vi "AVS Names to List.vi"(8 "error in":errorcluster, 11 "AVS names":T1) -> (0 "error out":errorcluster, 3 "List":string)   [LabVIEW 2019, in "Inst.TC.lvclass"]
uses:
  Inst.TC.lvclass
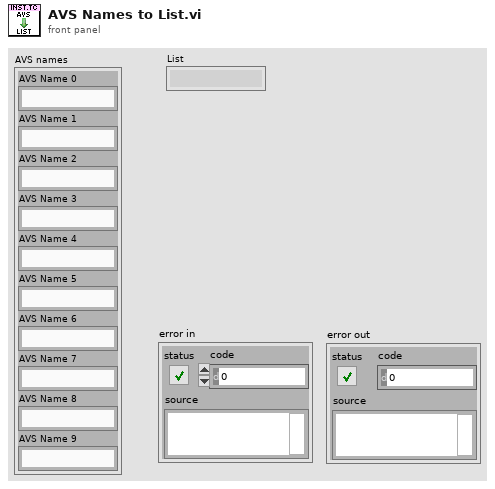
[diagram p1: front panel]
types:
  T1 = cluster{"AVS Name 0":string, "AVS Name 1":string, "AVS Name 2":string, "AVS Name 3":string, "AVS Name 4":string, "AVS Name 5":string, "AVS Name 6":string, "AVS Name 7":string, "AVS Name 8":string, "AVS Name 9":string}
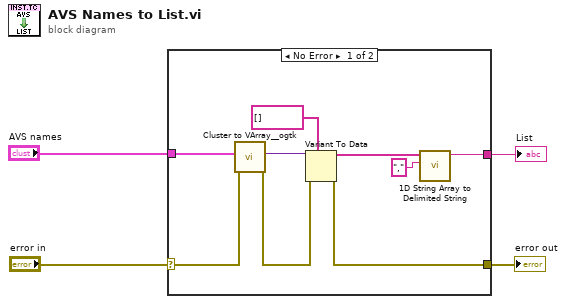
[diagram p0: block diagram]
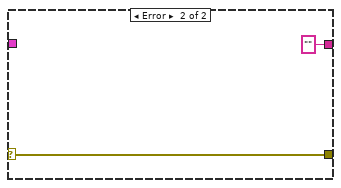
[diagram p2: hidden frame]
diagram:
  n1 = case shown="No Error" "error in" {
    selector: "error in" -> [w5 w15]
    tunnel: "AVS names" -> [w10 _]
    tunnel: [w9 "" ("delimited string")] -> w3
    tunnel: [w6 w15] -> w2
    frame No Error {
      n2 = call <userlib>:"Cluster to VArray__ogtk.vi"("error in (no error)"=w5, "Cluster"=w10) -> ("error out"=w7:errorcluster, "VArray"=w11:variant)  [unwired: 8 in]
      n3 = Variant To Data(error in=w7, type=string[] [], Variant=w11) -> (data=w12:string[], error out=w6:errorcluster)
      n4 = call <vilib>:"1D String Array to Delimited String.vi"("delimiter"=",", "string array"=w12) -> ("delimited string"=w9:string)  [unwired: 9 in]
    }
    frame Error {
    }
  }
  "List" <- w3
  "error out" <- w2
